vi "UTC.vi"(8 "error in (no error)":errorcluster) -> (0 "error out":errorcluster)   [LabVIEW 2014, in "MASTTCSGET.lvlib"]
doc: "this is the universal time\n\n\n__declspec (dllexport) float UTC();"
uses:
  MASTTCSGET.lvlib
  MASTTCSGET.dll
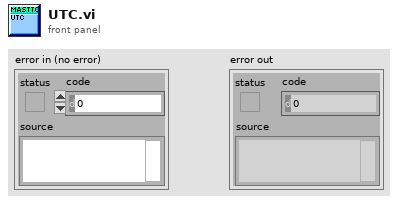
[diagram p1: front panel]
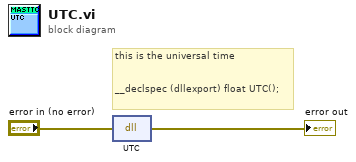
[diagram p0: block diagram]
diagram:
  # "this is the universal time\n\n\n__declspec (dllexport) float UTC();"
  n1 = dll-call lib="C:/Users/sanjay/Desktop/mast_controlsystem/MASTTCSGET.*" fn="UTC"(error in="error in (no error)") -> (error out=→"error out":errorcluster)  [unwired: 3 in, 1 out]
